vi "SPI.vi"() -> ()   [LabVIEW 2024]
uses:
  SPI_client.dll
panel:
  out "Progress":dbl(slide) scale=0.0..1.0
  in  "Wait [ms]":u32
  in  "Gray level of \"1\"":u32
  in  "Magnification factor":u32
  in  "Pattern size (power of two)":u32
  in  "Monitor No.":u32
  in  "Path to exe":path
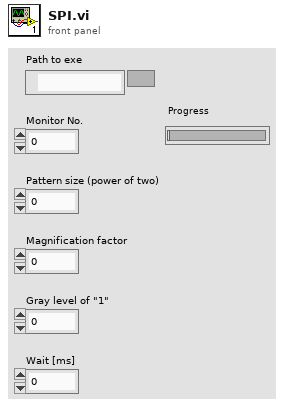
[diagram p1: front panel]
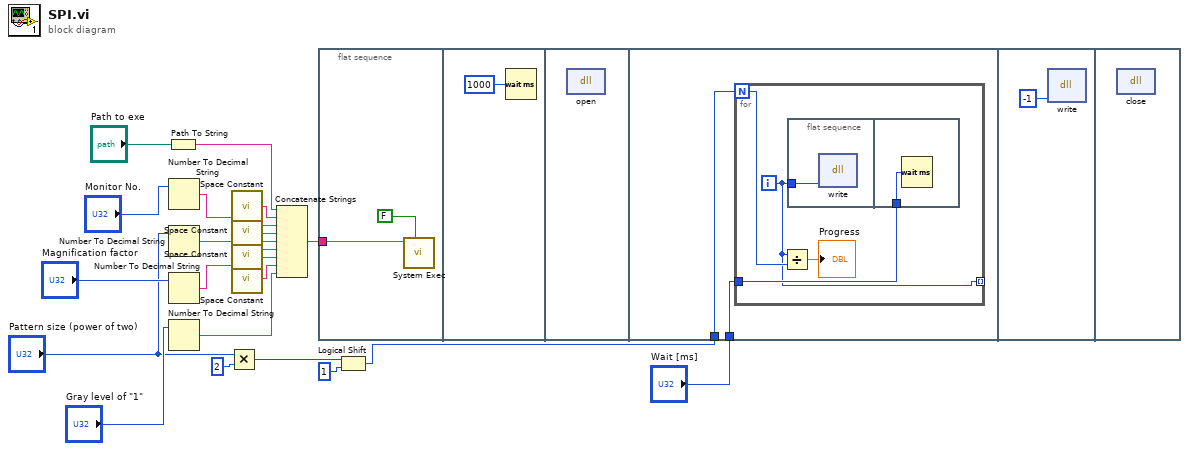
[diagram p0: block diagram]
diagram:
  n1 = Path To String(path="Path to exe") -> (string=w16:string)
  n2 = Number To Decimal String(number="Monitor No.") -> (decimal integer string=w14:string)  [unwired: 1 in]
  n3 = Number To Decimal String(number="Pattern size (power of two)") -> (decimal integer string=w12:string)  [unwired: 1 in]
  n4 = Number To Decimal String(number="Magnification factor") -> (decimal integer string=w10:string)  [unwired: 1 in]
  n5 = Number To Decimal String(number="Gray level of \"1\"") -> (decimal integer string=w8:string)  [unwired: 1 in]
  n6 = Multiply(x="Pattern size (power of two)", y=u32 2) -> (x*y=w2:u32)
  n7 = call <vilib>:"Space Constant.vi"() -> ("String"=w15:string)
  n8 = call <vilib>:"Space Constant.vi"() -> ("String"=w13:string)
  n9 = call <vilib>:"Space Constant.vi"() -> ("String"=w11:string)
  n10 = call <vilib>:"Space Constant.vi"() -> ("String"=w9:string)
  n11 = Concatenate Strings(w16, w15, w14, w13, w12, w11, w10, w9, w8) -> (w7:string)
  n12 = flat-sequence {
    tunnel: w7 -> [w22]
    tunnel: w1 -> [w25]
    tunnel: "Wait [ms]" -> [w24]
    frame #0 {
      n13 = call <vilib>:"System Exec.vi"("wait until completion? (T)"=FALSE, "command line"=w22) -> ()  [unwired: 6 in, 4 out]
    }
    frame #1 {
      n14 = Wait (ms)(milliseconds to wait=1000) -> ()  [unwired: 1 out]
    }
    frame #2 {
      n15 = dll-call lib="C:/Users/PhotonicsLab/Desktop/SPI/SPI_client.dll" fn="open"() -> ()  [unwired: 4 in, 2 out]
    }
    frame #3 {
      n16 = for {
        N: w25 -> [w27]
        tunnel: w24 -> [w29]
        tunnel: [w26] -> _ mode=indexing
        i -> [w26]
        n17 = Divide(x=w26, y=w27) -> (x/y=→"Progress":dbl)
        n18 = flat-sequence {
          tunnel: w26 -> [w30]
          tunnel: w29 -> [w31]
          frame #0 {
            n19 = dll-call lib="C:/Users/PhotonicsLab/Desktop/SPI/SPI_client.dll" fn="write"("arg1"=w30) -> ()  [unwired: 5 in, 2 out]
          }
          frame #1 {
            n20 = Wait (ms)(milliseconds to wait=w31) -> ()  [unwired: 1 out]
          }
        }
      }
    }
    frame #4 {
      n21 = dll-call lib="C:/Users/PhotonicsLab/Desktop/SPI/SPI_client.dll" fn="write"("arg1"=-1) -> ()  [unwired: 5 in, 2 out]
    }
    frame #5 {
      n22 = dll-call lib="C:/Users/PhotonicsLab/Desktop/SPI/SPI_client.dll" fn="close"() -> ()  [unwired: 4 in, 2 out]
    }
  }
  n23 = Logical Shift(y=w2, x=1) -> (x << y=w1:i32)
